vi "PipBoy_SendCommandToLabVIEW.vi"(8 "error in (no error)":errorcluster, 10 "Command":string, 11 "PipBoyDataIn":T1) -> (0 "error out":errorcluster)   [LabVIEW 2014]
uses:
  ctls/PipBoy_PipBoyData.ctl
  ctls/PipBoy_ProcComm.ctl
  System.Windows.Forms
  ctls/PipBoy_PipBoyCommand.ctl
  ctls/PipBoy_Message.ctl
  modules/support/Message Queue/All Message Queues.ctl
  modules/support/Message Queue/Message Cluster.ctl
  ctls/PipBoy_FileConf.ctl
  ctls/PipBoy_PicComm.ctl
  ctls/PipBoy_GeneralParams.ctl
  ctls/PipBoy_Pages.ctl
  modules/support/Message Queue/Message Queue.lvlib
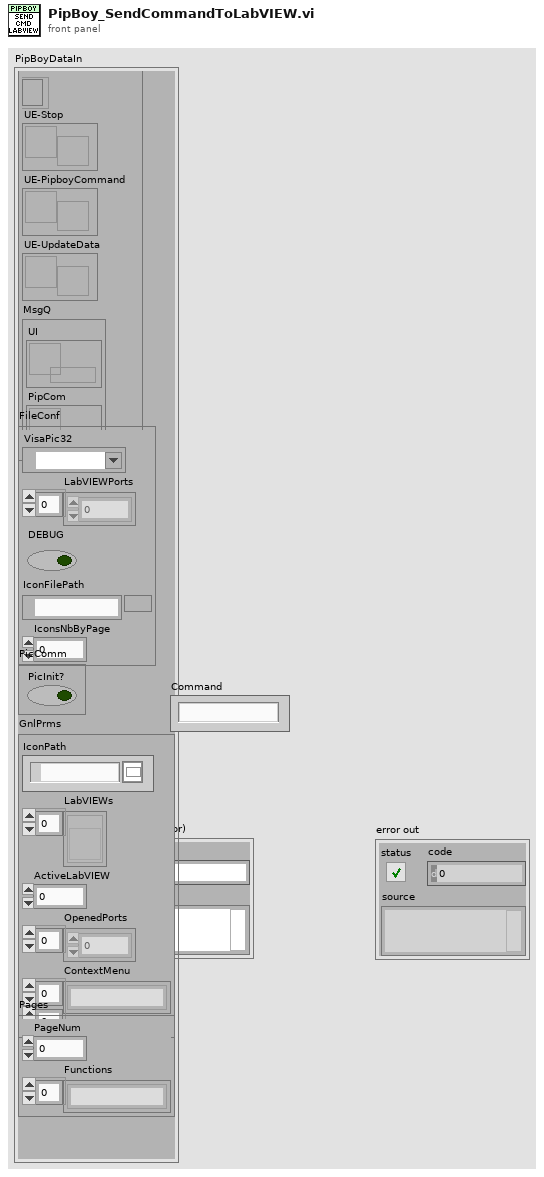
[diagram p1: front panel]
types:
  T1 = typedef "PipBoy_PipBoyData.ctl" = cluster{"ProcComm":T2, "FileConf":T4, "PicComm":T5, "GnlPrms":T6, "Pages":T7}
  T2 = typedef "PipBoy_ProcComm.ctl" = cluster{"NotifyIconRef":refnum<k24>, "UE-Stop":refnum<user-event>, "UE-PipboyCommand":refnum<user-event>, "UE-UpdateData":refnum<user-event>, "MsgQ":T3}
  T3 = typedef "Message Queue.lvlib/All Message Queues.ctl" = cluster{"UI":refnum<queue>, "PipCom":refnum<queue>}
  T4 = typedef "PipBoy_FileConf.ctl" = cluster{"VisaPic32":refnum<visa-resource-name>, "LabVIEWPorts":u16[], "DEBUG":bool, "IconFilePath":path, "IconsNbByPage":i32}
  T5 = typedef "PipBoy_PicComm.ctl" = cluster{"PicInit?":bool}
  T6 = typedef "PipBoy_GeneralParams.ctl" = cluster{"IconPath":path, "LabVIEWs":refnum<vi>[], "ActiveLabVIEW":i32, "OpenedPorts":u16[], "ContextMenu":string[][]}
  T7 = typedef "PipBoy_Pages.ctl" = cluster{"PageNum":i32, "Functions":string[]}
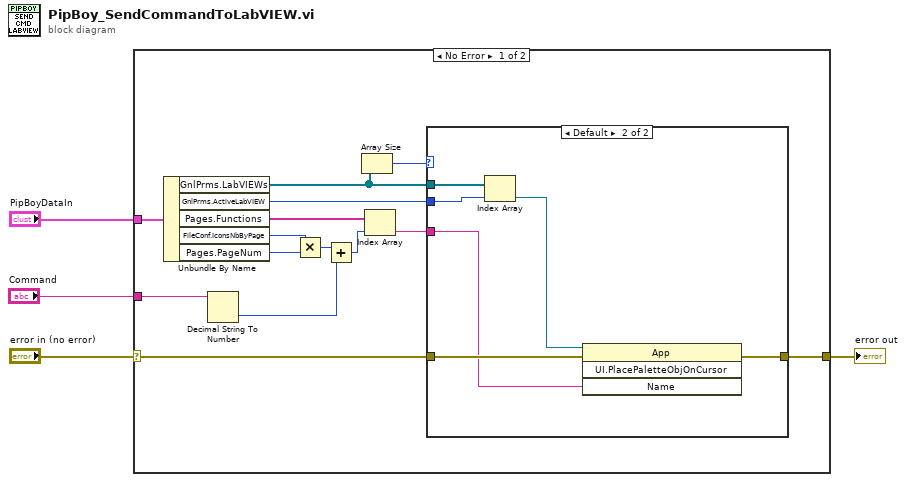
[diagram p0: block diagram]
diagram:
  n1 = case shown="No Error" "error in (no error)" {
    selector: "error in (no error)" -> [w16 w26]
    tunnel: [w17 w26] -> w3
    tunnel: "PipBoyDataIn" -> [w18 _]
    tunnel: "Command" -> [w12 _]
    frame No Error {
      n2 = Unbundle By Name(w18) -> ("GnlPrms.LabVIEWs"=w15:refnum<vi>[], "GnlPrms.ActiveLabVIEW"=w13:i32, "Pages.Functions"=w11:string[], "FileConf.IconsNbByPage"=w9:i32, "Pages.PageNum"=w8:i32)
      n3 = Decimal String To Number(string=w12) -> (number=w6:i32)  [unwired: 2 in, 1 out]
      n4 = Multiply(x=w9, y=w8) -> (x*y=w7:i32)
      n5 = Add(x=w7, y=w6) -> (x+y=w5:i32)
      n6 = Array Size(array=w15) -> (size(s)=w14:i32)
      n7 = Index Array(array=w11, index=w5) -> (element=w10:string)
      n8 = case shown="Default" w14 {
        tunnel: [w19 w21] -> w17
        tunnel: w16 -> [w19 w23]
        tunnel: w15 -> [_ w25]
        tunnel: w13 -> [_ w24]
        tunnel: w10 -> [_ w20]
        frame ..0 {
        }
        frame Default {
          n9 = Index Array(array=w25, index=w24) -> (element=w22:refnum<vi>)
          n10 = invoke class="App" method="UI.PlacePaletteObjOnCursor"(reference=w22, error in=w23, "Name"=w20) -> (error out=w21:errorcluster)  [unwired: 1 in, 3 out]
        }
      }
    }
    frame Error {
    }
  }
  "error out" <- w3
